vi "NT Format Generic  to String.vi"(9 "Quote Elements":bool, 11 "Field Value":T1) -> (3 "String":string)   [LabVIEW 2017]
doc: "Format the generic union data into a string."
uses:
  <vilib>/Rock Robotics/Network Tables/Field Data.ctl
  <vilib>/Rock Robotics/Network Tables/Field Type.ctl
  <vilib>/Rock Robotics/Network Tables/Sequence.ctl
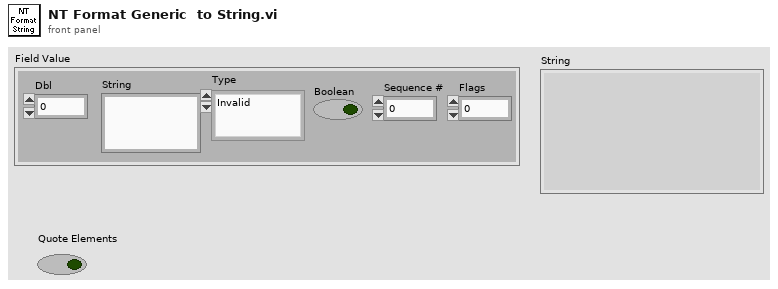
[diagram p1: front panel]
types:
  T1 = typedef "Field Data.ctl" = cluster{"Dbl":dbl, "String":string, "Type":T2, "Boolean":bool, "Sequence #":T3, "Flags":u8}
  T2 = typedef "Field Type.ctl" = enum8{"Invalid", "Bool", "Numeric", "String", "Raw", "Boolean Array", "Numeric Array", "String Array", "RPC"}
  T3 = typedef "Sequence.ctl" = u16
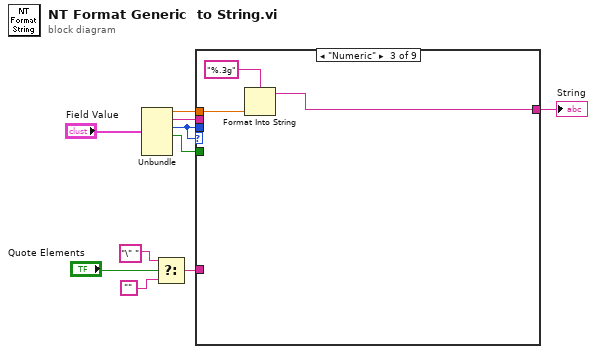
[diagram p0: block diagram]
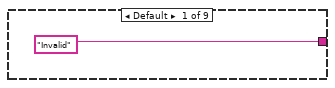
[diagram p2: hidden frame]
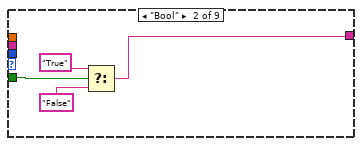
[diagram p3: hidden frame]
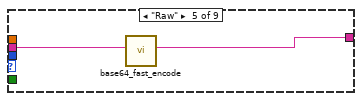
[diagram p5: hidden frame]
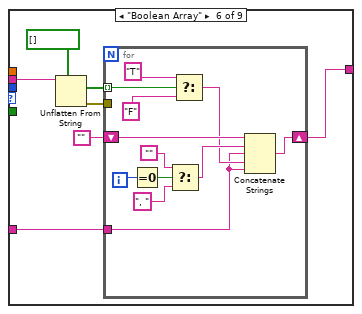
[diagram p6: hidden frame]
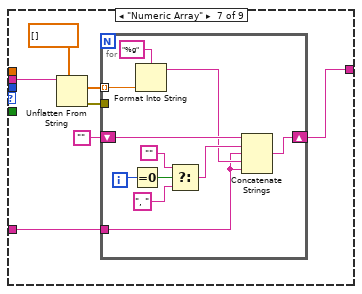
[diagram p7: hidden frame]
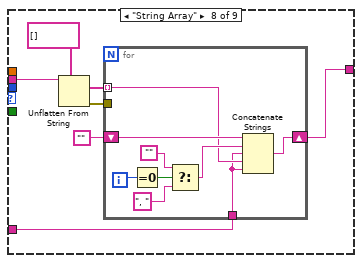
[diagram p8: hidden frame]
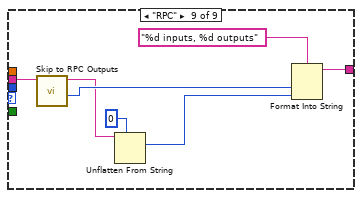
[diagram p9: hidden frame]
diagram:
  n1 = Unbundle("Field Value") -> ("Dbl"=w9:dbl, "String"=w8:string, "Type"=w6:T2, "Boolean"=w5:bool)  [unwired: 2 out]
  n2 = Select(t="\" ", s="Quote Elements", f="") -> (s? t:f=w1:string)
  n3 = case shown="\"Numeric\"" w6 {
    tunnel: w5 -> [_ w13 _ _ _ _ _ _ _]
    tunnel: w6 -> [_ _ _ _ _ _ _ _ _]
    tunnel: w8 -> [_ _ _ w19 w21 w27 w47 w65 w79]
    tunnel: w9 -> [_ _ w18 _ _ _ _ _ _]
    tunnel: ["Invalid" w12 w17 w19 w20 w24 w44 w62 w81] -> w10
    tunnel: w1 -> [_ _ _ _ _ w22 w41 w59 _]
    frame Default {
    }
    frame "Bool" {
      n4 = Select(t="True", s=w13, f="False") -> (s? t:f=w12:string)
    }
    frame "Numeric" {
      n5 = Format Into String(format string="%.3g", w18) -> (resulting string=w17:string)  [unwired: 2 in, 1 out]
    }
    frame "String" {
    }
    frame "Raw" {
      n6 = call <vilib>:"base64_fast_encode.vi"("string in (not encoded)"=w21) -> ("string out (base64-encoded)"=w20:string)  [unwired: 9 in, 1 out]
    }
    frame "Boolean Array" {
      n7 = Unflatten From String(type=bool[] [], binary string=w27) -> (value=w26:bool[], error out=w23:errorcluster)  [unwired: 3 in, 1 out]
      n8 = for {
        tunnel: w26 -> [w38] mode=indexing
        shift-right: [w31] -> w24
        shift-left: "" -> [w37]
        tunnel: w23 -> [_]
        tunnel: w22 -> [w29]
        i -> [w36]
        n9 = Equal To 0?(x=w36) -> (x = 0?=w35:bool)
        n10 = Select(t="", s=w35, f=", ") -> (s? t:f=w32:string)
        n11 = Select(t="T", s=w38, f="F") -> (s? t:f=w30:string)
        n12 = Concatenate Strings(w37, w32, w29, w30, w29) -> (w31:string)
      }
    }
    frame "Numeric Array" {
      n13 = Unflatten From String(type=dbl[] [], binary string=w47) -> (value=w46:dbl[], error out=w42:errorcluster)  [unwired: 3 in, 1 out]
      n14 = for {
        tunnel: w46 -> [w51] mode=indexing
        shift-right: [w52] -> w44
        shift-left: "" -> [w58]
        tunnel: w42 -> [_]
        tunnel: w41 -> [w48]
        i -> [w57]
        n15 = Equal To 0?(x=w57) -> (x = 0?=w56:bool)
        n16 = Format Into String(format string="%g", w51) -> (resulting string=w49:string)  [unwired: 2 in, 1 out]
        n17 = Select(t="", s=w56, f=", ") -> (s? t:f=w53:string)
        n18 = Concatenate Strings(w58, w53, w48, w49, w48) -> (w52:string)
      }
    }
    frame "String Array" {
      n19 = Unflatten From String(type=string[] [], binary string=w65) -> (value=w64:string[], error out=w60:errorcluster)  [unwired: 3 in, 1 out]
      n20 = for {
        tunnel: w64 -> [w67] mode=indexing
        shift-right: [w68] -> w62
        shift-left: "" -> [w74]
        tunnel: w60 -> [_]
        tunnel: w59 -> [w66]
        i -> [w73]
        n21 = Equal To 0?(x=w73) -> (x = 0?=w72:bool)
        n22 = Select(t="", s=w72, f=", ") -> (s? t:f=w69:string)
        n23 = Concatenate Strings(w74, w69, w66, w67, w66) -> (w68:string)
      }
    }
    frame "RPC" {
      n24 = call <vilib>:"Skip to RPC Outputs.vi"("String in"=w79) -> ("inputs"=w78:u8, "String out"=w76:string)  [unwired: 8 in, 1 out]
      n25 = Unflatten From String(type=u8 0 ("bytes to read"), binary string=w76) -> (value=w75:u8)  [unwired: 3 in, 2 out]
      n26 = Format Into String(format string="%d inputs, %d outputs", w78, w75) -> (resulting string=w81:string)  [unwired: 2 in, 1 out]
    }
  }
  "String" <- w10
